vi "Write Ramp Rate.vi"(8 "error in (no error)":errorcluster, 10 "Ramp Rate [degC/s]":dbl, 11 "Thermal Chamber Response Simlator in":refnum<class "Thermal Chamber Response Simlator.lvclass">) -> (0 "error out":errorcluster, 3 "Thermal Chamber Response Simlator out":refnum<class "Thermal Chamber Response Simlator.lvclass">)   [LabVIEW 2020, in "Thermal Chamber Response Simlator.lvclass"]
uses:
  Thermal Chamber Response Simlator.lvclass
  Thermal Chamber Response Simlator.lvclass/Thermal Chamber Response Simlator.ctl
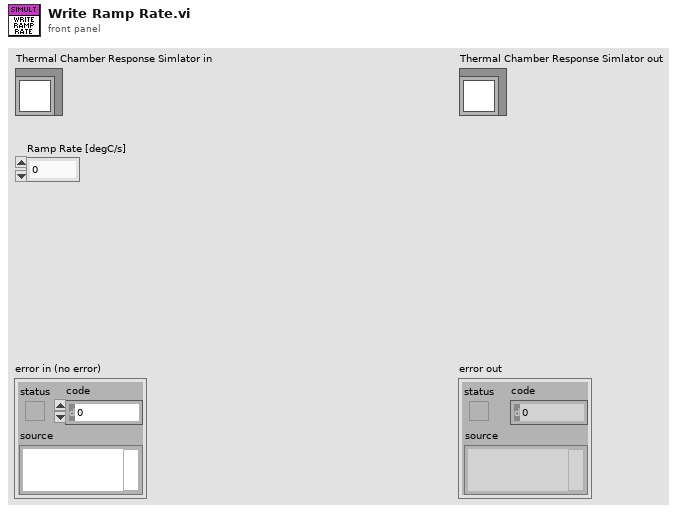
[diagram p1: front panel]
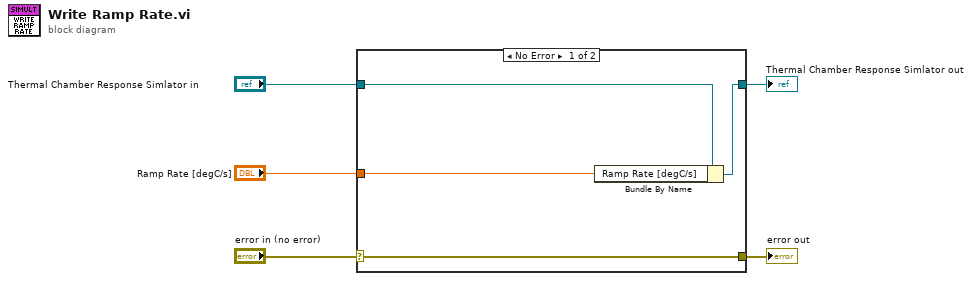
[diagram p0: block diagram]
diagram:
  n1 = case shown="No Error" "error in (no error)" {
    selector: "error in (no error)" -> [w9 w10]
    tunnel: [w9 w10] -> w4
    tunnel: [w7 w11] -> w2
    tunnel: "Thermal Chamber Response Simlator in" -> [w8 w11]
    tunnel: "Ramp Rate [degC/s]" -> [w6 _]
    frame No Error {
      n2 = Bundle By Name(cluster=w8, "Ramp Rate [degC/s]"=w6) -> (w7:refnum<class "Thermal Chamber Response Simlator.lvclass">)
    }
    frame Error {
    }
  }
  "error out" <- w4
  "Thermal Chamber Response Simlator out" <- w2
